vi "test.vi"() -> ()   [LabVIEW 2018]
uses:
  <vilib>/Utility/file.llb/Read Delimited Spreadsheet (DBL).vi
panel:
  out "Массив в формате boolean":bool[][](array[boolean])
  out "Массив регистров":string[][](array[string])
  out "array":i32[](array[numeric])
  out "Array":string[](array[string])
  out "Начальные данные":dbl[][](array[numeric])
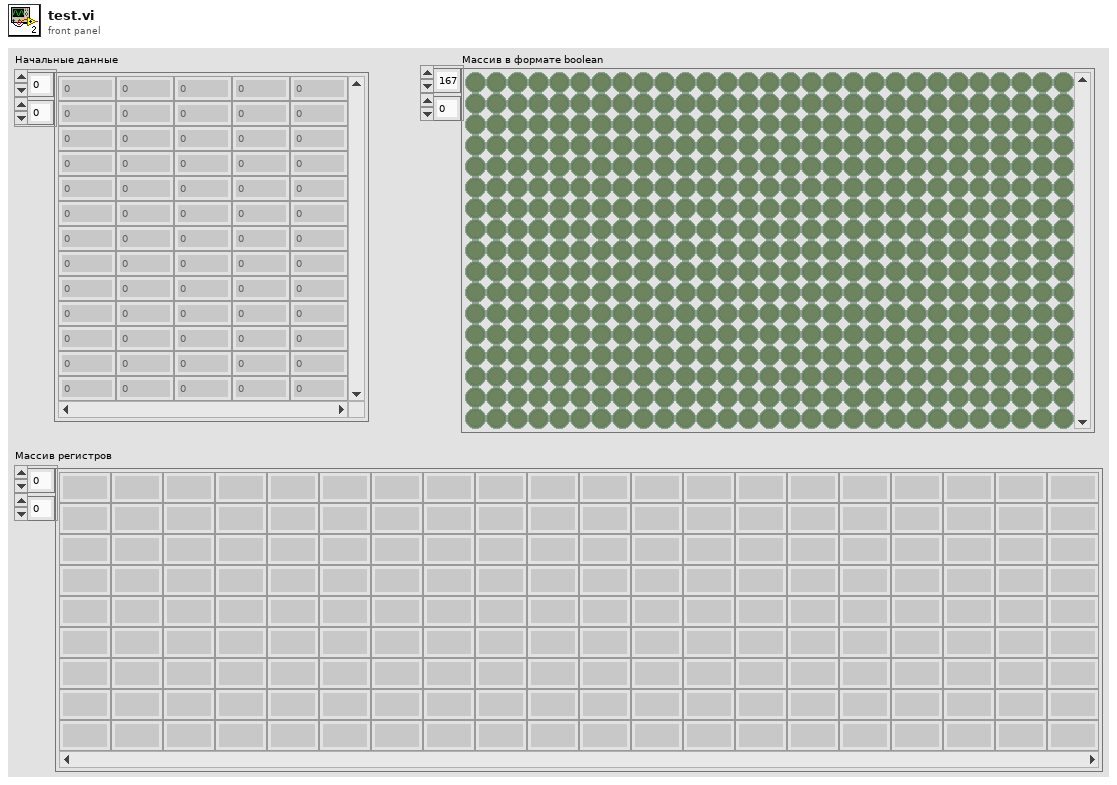
[diagram p1: front panel]
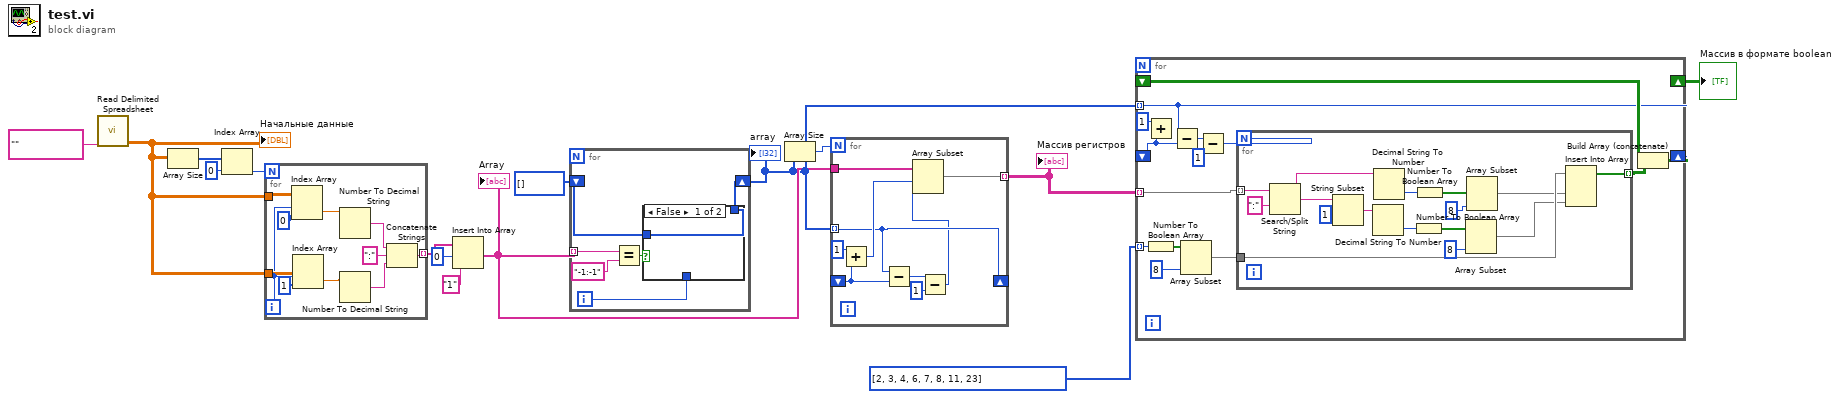
[diagram p0: block diagram]
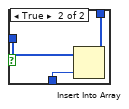
[diagram p2: hidden frame]
diagram:
  n1 = call-poly <vilib>:"Read Delimited Spreadsheet.vi"("delimiter (\\t)"="" ("delimiter (\\t)")) -> ("all rows"=w14:dbl[][])  [unwired: 9 in, 5 out]
  "Начальные данные" <- w14
  n2 = Array Size(array=w14) -> (size(s)=w13:i32[])
  n3 = Index Array(array=w13, index=0) -> (element=w11:i32)
  n4 = for {
    N: w11 -> [_]
    tunnel: w14 -> [w26]
    tunnel: w14 -> [w22]
    tunnel: [w20] -> w9 mode=indexing
    i -> [w21]
    n5 = Index Array(array=w22, index (row)=w21, index (col)=0 ("disabled index (col)")) -> (element=w17:dbl)
    n6 = Index Array(array=w26, index (row)=w21, index (col)=1 ("disabled index (col)")) -> (element=w16:dbl)
    n7 = Number To Decimal String(number=w17) -> (decimal integer string=w25:string)  [unwired: 1 in]
    n8 = Number To Decimal String(number=w16) -> (decimal integer string=w24:string)  [unwired: 1 in]
    n9 = Concatenate Strings(w25, ":" ("string"), w24) -> (w20:string)
  }
  n10 = Insert Into Array(array=w9, index=0, new element="1" ("new element/subarray")) -> (w6:string[])
  "Array" <- w6
  n11 = for {
    tunnel: w6 -> [w31] mode=indexing
    shift-right: [w27] -> w1
    shift-left: i32[] [] ("array") -> [w28]
    i -> [w29]
    n12 = Equal?(x=w31, y="-1:-1") -> (x = y?=w30:bool)
    n13 = case shown="False" w30 {
      tunnel: w29 -> [_ w36]
      tunnel: w28 -> [w33 w35]
      tunnel: [w33 w34] -> w27
      frame False {
      }
      frame True {
        n14 = Insert Into Array(array=w35, new element=w36) -> (w34:i32[])  [unwired: 1 in]
      }
    }
  }
  "array" <- w1
  n15 = Array Size(array=w1) -> (size(s)=w3:i32)
  n16 = for {
    N: w3 -> [_]
    tunnel: w1 -> [w40] mode=indexing
    tunnel: w6 -> [w45]
    shift-right: [w40] -> _
    shift-left: _ -> [w43]
    tunnel: [w44] -> w5 mode=indexing
    n17 = Add(x=1, y=w43) -> (x+y=w41:i32)
    n18 = Subtract(x=w40, y=w43) -> (x-y=w39:i32)
    n19 = Subtract(x=w39, y=1) -> (x-y=w38:i32)
    n20 = Array Subset(array=w45, index=w41, length=w38) -> (w44:string[])
  }
  "Массив регистров" <- w5
  n21 = for {
    tunnel: w5 -> [w54] mode=indexing
    tunnel: i32[] [2, 3, 4, 6, 7, 8, 11, 23] -> [w59] mode=indexing
    shift-right: [w52] -> w2
    shift-left: _ -> [w53]
    tunnel: w1 -> [w47] mode=indexing
    shift-right: [w47] -> _
    shift-left: _ -> [w46]
    n22 = Add(x=1, y=w46) -> ()  [unwired: 1 out]
    n23 = Number To Boolean Array(number=w59) -> (Boolean array=w56:bool[])
    n24 = Subtract(x=w47, y=w46) -> (x-y=w51:i32)
    n25 = Array Subset(array=w56, length=8) -> (w57:bool[])  [unwired: 1 in]
    n26 = Subtract(x=w51, y=1) -> (x-y=w49:i32)
    n27 = for {
      N: w49 -> [_]
      tunnel: w54 -> [w74] mode=indexing
      tunnel: w57 -> [w66]
      tunnel: [w67] -> w58 mode=indexing
      n28 = Search/Split String(string=w74, search string/char (-)=":") -> (substring before match=w68:string, match + rest of string=w73:string)  [unwired: 1 in, 1 out]
      n29 = String Subset(string=w73, offset (0)=1) -> (substring=w71:string)  [unwired: 1 in]
      n30 = Decimal String To Number(string=w71) -> (number=w70:i32)  [unwired: 2 in, 1 out]
      n31 = Decimal String To Number(string=w68) -> (number=w69:i32)  [unwired: 2 in, 1 out]
      n32 = Number To Boolean Array(number=w70) -> (Boolean array=w65:bool[])
      n33 = Number To Boolean Array(number=w69) -> (Boolean array=w64:bool[])
      n34 = Array Subset(array=w65, length=8) -> (w60:bool[])  [unwired: 1 in]
      n35 = Array Subset(array=w64, length=8) -> (w61:bool[])  [unwired: 1 in]
      n36 = Insert Into Array(array=w66, new element #1=w61, new element #2=w60) -> (w67:bool[])  [unwired: 1 in]
    }
    n37 = Build Array (concatenate)(w53, w58) -> (w52:bool[][])
  }
  "Массив в формате boolean" <- w2
